vi "Wait.vi"(6 "ms":u32, 7 "Error In":errorcluster) -> (3 "Error Out":errorcluster)   [LabVIEW 2020, in "Endigit.lvlib"]
doc: "Waits the number of specified milliseconds. This VI is designed to allow the error terminals to specify order of operations.\n\nAuthored by Robert C. Mortensen\nrobert@endigit.com\n\nCopyright (c) 2015, Endigit, Inc."
uses:
  Endigit.lvlib
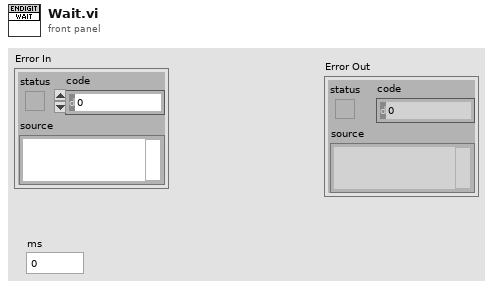
[diagram p1: front panel]
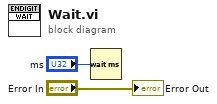
[diagram p0: block diagram]
diagram:
  n1 = Wait (ms)(milliseconds to wait="ms") -> ()  [unwired: 1 out]
  "Error Out" <- "Error In"
